vi "TestExec.Configure Local Station ID Read and Dialog.vi"(9 "Dialog":bool, 10 "Station":T1={"Name"="UNDEFINED", "PN"="UNDEFINED", "SN"="UNDEFINED", "Location"="UNDEFINED"}, 11 "Config File":path) -> (1 "Changed":bool, 3 "Station Out":T1)   [LabVIEW 2024]
uses:
  TestExec.Station ID.ctl
  <vilib>/Utility/config.llb/Read Key (String).vi
  <vilib>/Utility/config.llb/Write Key (String).vi
  <vilib>/Utility/config.llb/NI_LVConfig.lvlib
panel:
  out "Tab Control":enum32{"Inputs", "Data", "Outputs"}(tab)=enum."Data"
  in  "Default Sequence":u16(ring)
  in  "Additional Station  Config File":path
  in  "Changed":bool
  in  "Cancel":bool
  # "Local Station ID"
  # "(Optional)"
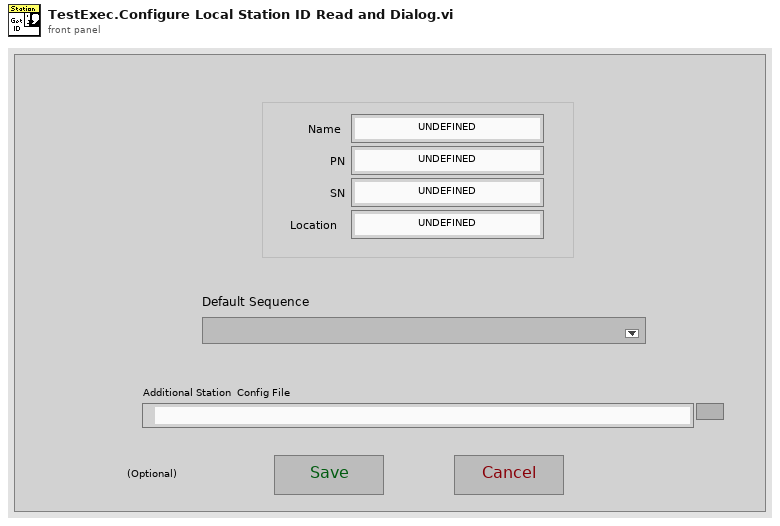
[diagram p1: front panel]
types:
  T1 = typedef "TestExec.Station ID.ctl" = cluster{"Name":string, "PN":string, "SN":string, "Location":string}
  T2 = enum32{"Invalid", "Standard", "Closed", "Hidden", "Minimized", "Maximized"}
  T3 = cluster{"Config File":path, "Changed":bool, "SeqDir":path}
  T4 = typedef "NI_LVConfig.lvlib/Config Data RefNum.ctl" = refnum<k1>
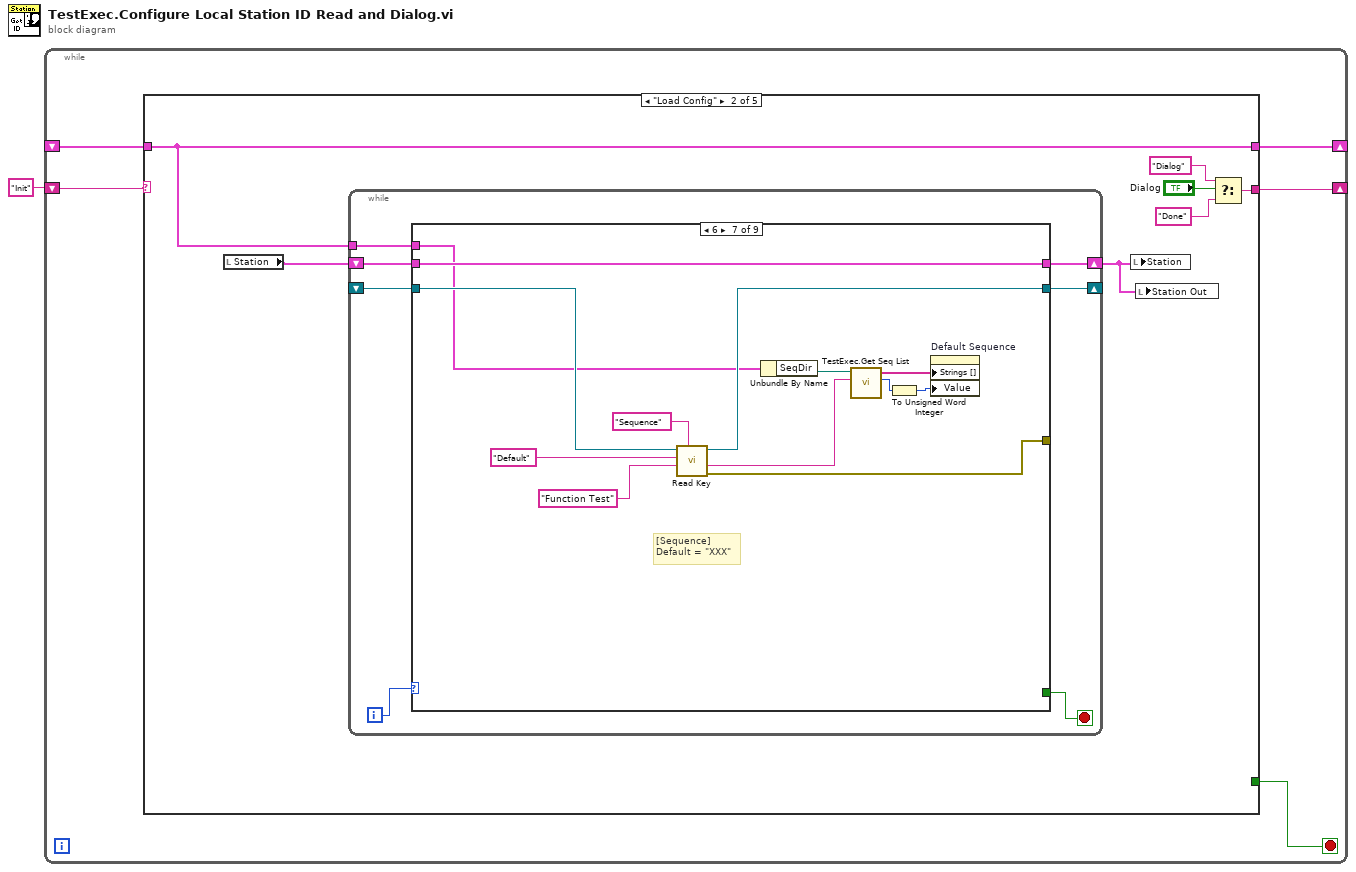
[diagram p0: block diagram]
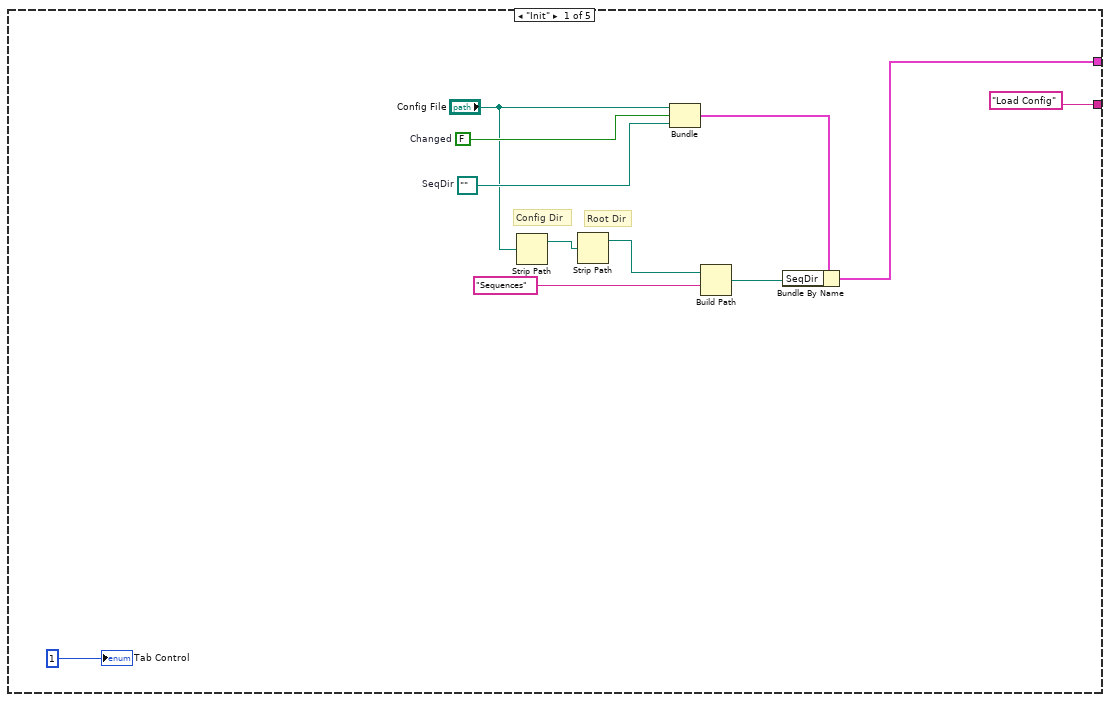
[diagram p2: hidden frame]
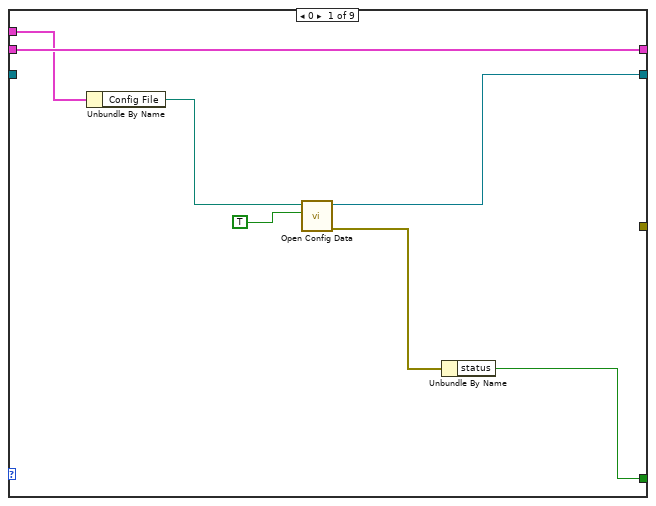
[diagram p3: hidden frame]
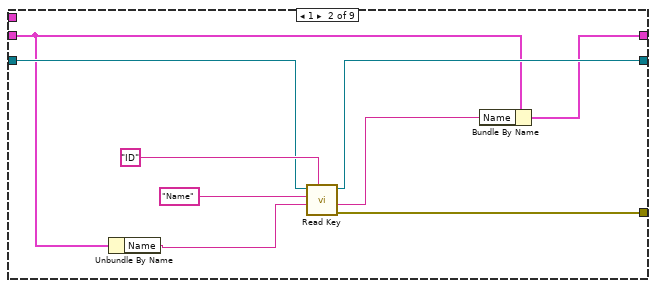
[diagram p4: hidden frame]
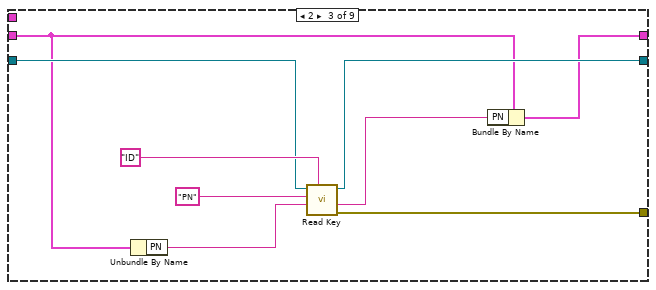
[diagram p5: hidden frame]
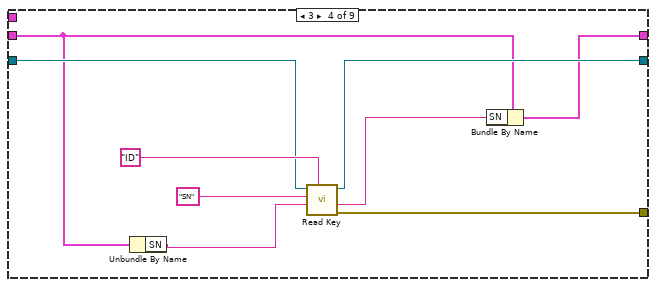
[diagram p6: hidden frame]
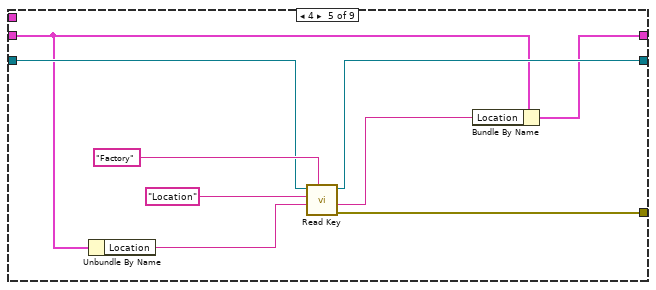
[diagram p7: hidden frame]
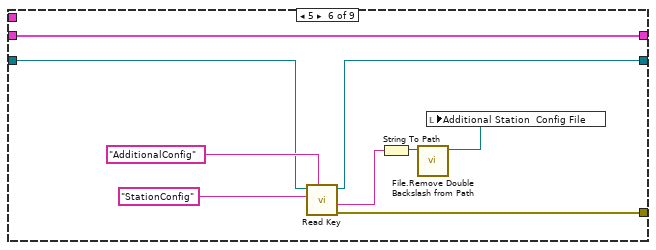
[diagram p8: hidden frame]
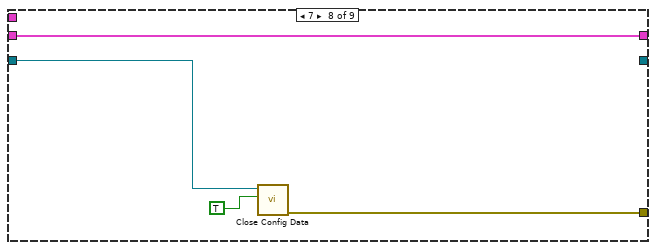
[diagram p9: hidden frame]
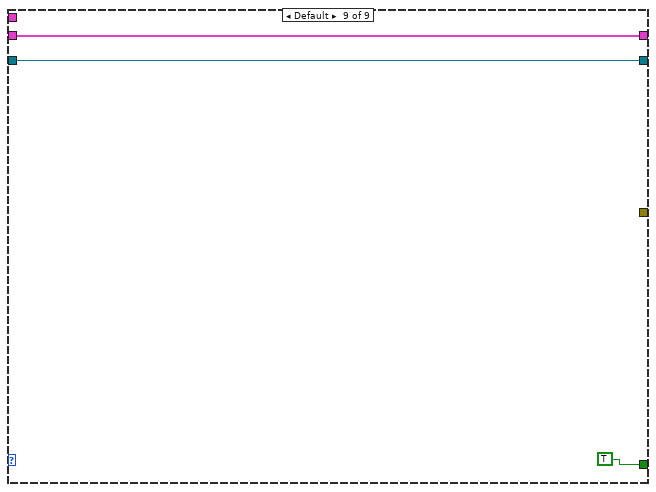
[diagram p10: hidden frame]
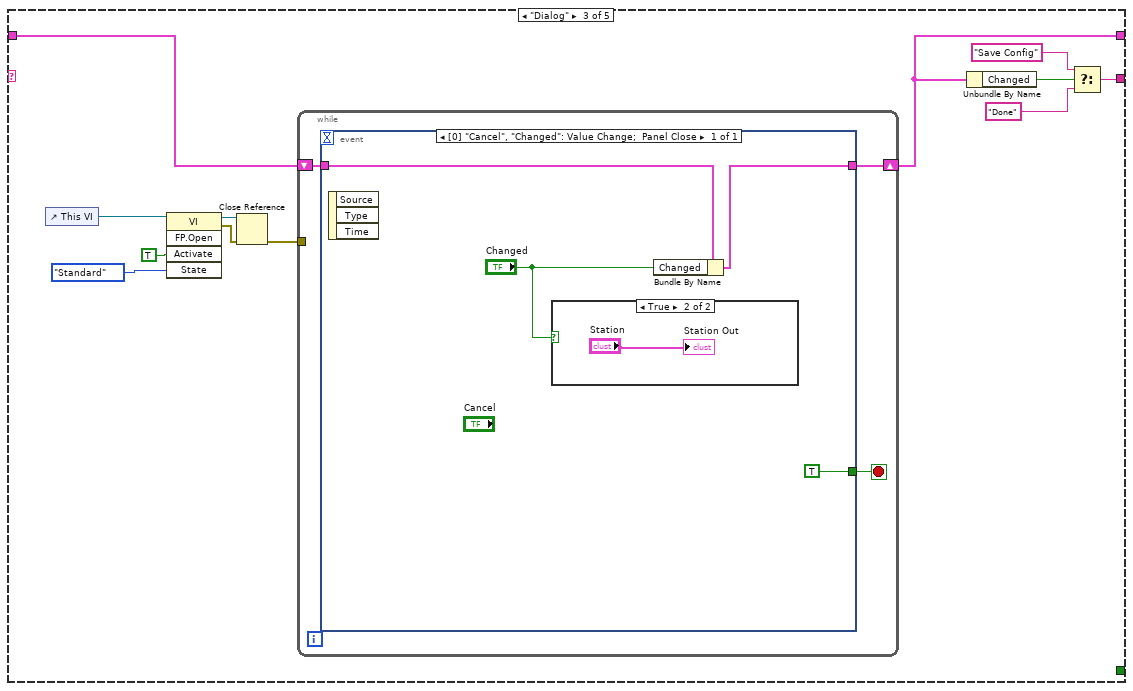
[diagram p11: hidden frame]
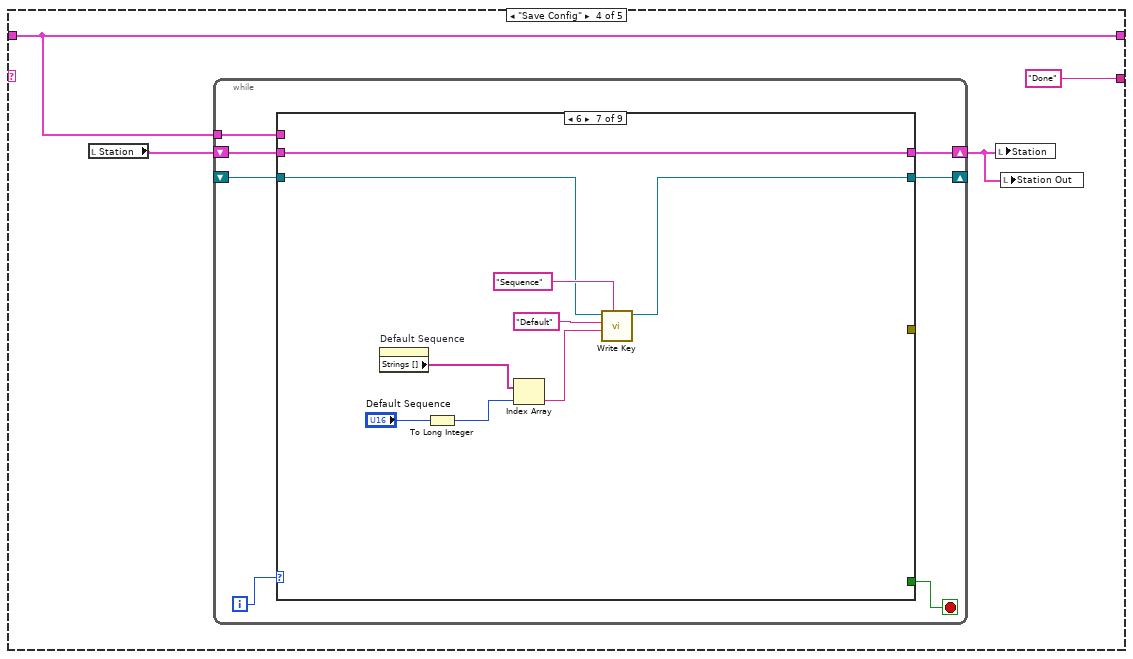
[diagram p13: hidden frame]
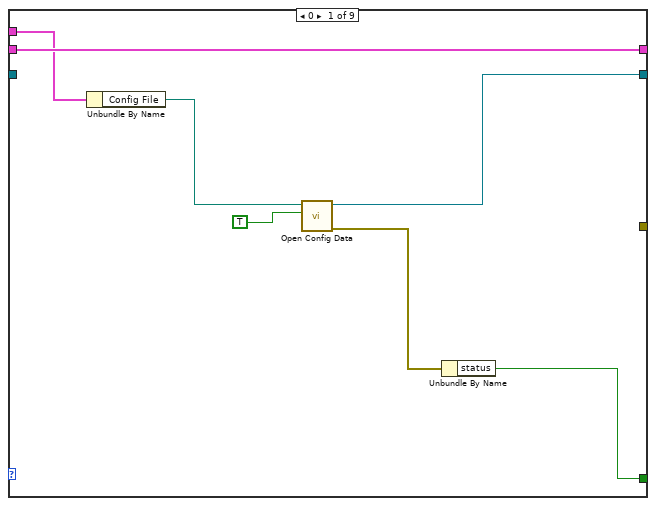
[diagram p14: hidden frame]
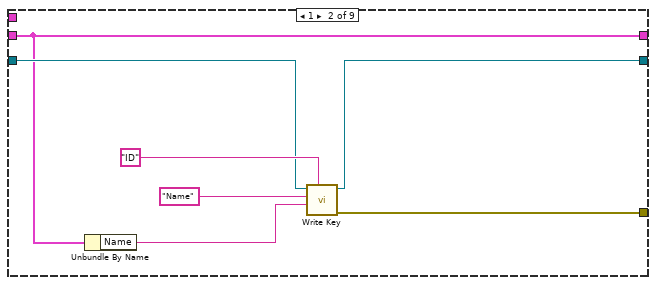
[diagram p15: hidden frame]
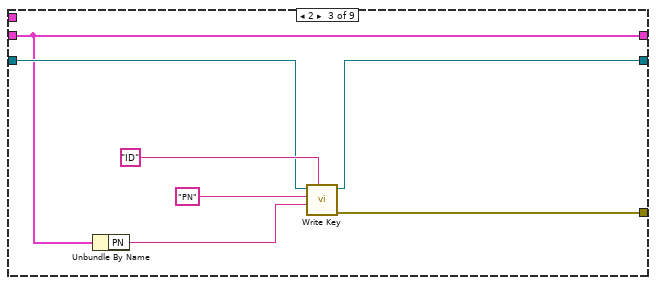
[diagram p16: hidden frame]
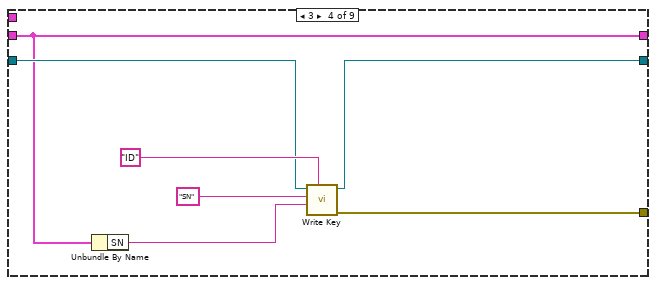
[diagram p17: hidden frame]
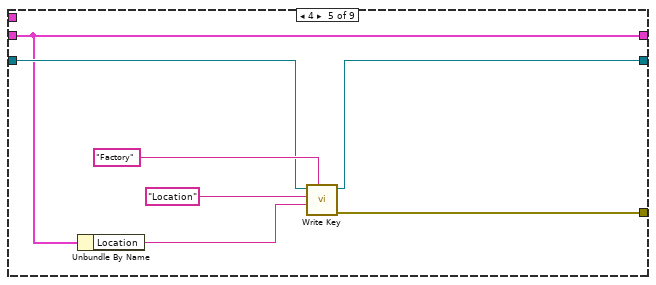
[diagram p18: hidden frame]
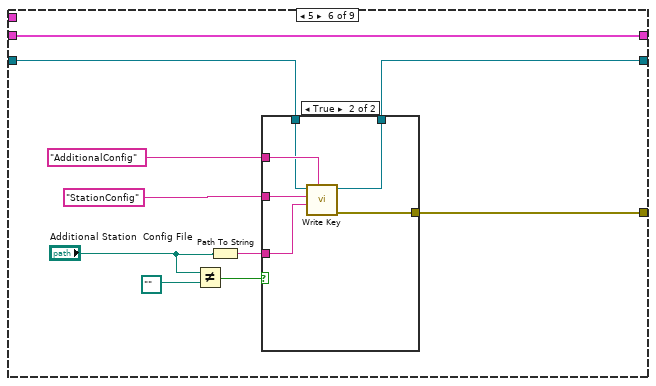
[diagram p19: hidden frame]
diagram:
  n1 = while {
    shift-right: [w4] -> _
    shift-left: _ -> [w6]
    shift-right: [w3] -> _
    shift-left: "Init" -> [w5]
    stop <- w2 stop-if-true
    n2 = case shown="\"Load Config\"" w5 {
      tunnel: w6 -> [_ w23 w109 w126 w207]
      tunnel: [w8 w23 w108 w126 w207] -> w4
      tunnel: ["Load Config" w21 w104 "Done" "Done"] -> w3
      tunnel: [_ _ _ _ TRUE] -> w2
      frame "Init" {
        w14 = path ""  # SeqDir
        w15 = FALSE  # Changed
        # "Root Dir"
        # "Config Dir"
        n3 = Strip Path(path="Config File") -> (stripped path=w11:path)  [unwired: 1 out]
        n4 = Strip Path(path=w11) -> (stripped path=w10:path)  [unwired: 1 out]
        n5 = Bundle("Config File"="Config File", "Changed"=w15, "SeqDir"=w14) -> (w9:T3)  [unwired: 1 in]
        n6 = Build Path(base path=w10, name or relative path="Sequences") -> (appended path=w7:path)
        n7 = Bundle By Name(cluster=w9, "SeqDir"=w7) -> (w8:T3)
        "Tab Control" <- 1
      }
      frame "Load Config" {
        n8 = local read "Station"() -> (w24:T1)
        n9 = while {
          shift-right: [w28] -> _
          shift-left: _ -> [w29]
          shift-right: [w27] -> w18
          shift-left: w24 -> [w26]
          tunnel: w23 -> [w25]
          i -> [w31]
          stop <- w30 stop-if-true
          n10 = case shown="6" w31 {
            tunnel: [w36 _ _ _ _ _ _ _ TRUE] -> w30
            tunnel: w29 -> [_ w44 w53 w62 w71 w80 w92 w100 w103]
            tunnel: [w38 w43 w52 w61 w70 w79 w93 _ w103] -> w28
            tunnel: [_ w47 w56 w65 w74 w83 w91 w99 _] -> _
            tunnel: [w34 w42 w51 w60 w69 w78 w96 w97 w102] -> w27
            tunnel: w26 -> [w34 w40 w49 w58 w67 w78 w96 w97 w102]
            tunnel: w25 -> [w33 _ _ _ _ _ w90 _ _]
            frame 0 {
              n11 = Unbundle By Name(w33) -> ("Config File"=w32:path)
              n12 = call <vilib>:"Open Config Data.vi"("create file if necessary (T)"=TRUE, "configuration file path"=w32) -> ("error out"=w37:errorcluster, "refnum"=w38:T4)  [unwired: 7 in, 1 out]
              n13 = Unbundle By Name(w37) -> ("status"=w36:bool)
            }
            frame 1 {
              n14 = Unbundle By Name(w40) -> ("Name"=w39:string)
              n15 = call-poly <vilib>:"Read Key.vi"("section"="ID", "default value"=w39, "key"="Name" ("section"), "refnum"=w44) -> ("error out"=w47:errorcluster, "value"=w41:string, "refnum out"=w43:T4)  [unwired: 4 in, 1 out]
              n16 = Bundle By Name(cluster=w40, "Name"=w41) -> (w42:T1)
            }
            frame 2 {
              n17 = Unbundle By Name(w49) -> ("PN"=w48:string)
              n18 = call-poly <vilib>:"Read Key.vi"("section"="ID", "default value"=w48, "key"="PN" ("section"), "refnum"=w53) -> ("error out"=w56:errorcluster, "value"=w50:string, "refnum out"=w52:T4)  [unwired: 4 in, 1 out]
              n19 = Bundle By Name(cluster=w49, "PN"=w50) -> (w51:T1)
            }
            frame 3 {
              n20 = Unbundle By Name(w58) -> ("SN"=w57:string)
              n21 = call-poly <vilib>:"Read Key.vi"("section"="ID", "default value"=w57, "key"="SN" ("section"), "refnum"=w62) -> ("error out"=w65:errorcluster, "value"=w59:string, "refnum out"=w61:T4)  [unwired: 4 in, 1 out]
              n22 = Bundle By Name(cluster=w58, "SN"=w59) -> (w60:T1)
            }
            frame 4 {
              n23 = Unbundle By Name(w67) -> ("Location"=w66:string)
              n24 = call-poly <vilib>:"Read Key.vi"("section"="Factory", "default value"=w66, "key"="Location" ("section"), "refnum"=w71) -> ("error out"=w74:errorcluster, "value"=w68:string, "refnum out"=w70:T4)  [unwired: 4 in, 1 out]
              n25 = Bundle By Name(cluster=w67, "Location"=w68) -> (w69:T1)
            }
            frame 5 {
              n26 = call-poly <vilib>:"Read Key.vi"("section"="AdditionalConfig", "key"="StationConfig" ("section"), "refnum"=w80) -> ("error out"=w83:errorcluster, "value"=w77:string, "refnum out"=w79:T4)  [unwired: 5 in, 1 out]
              n27 = String To Path(string=w77) -> (path=w76:path)
              n28 = call "File.Remove Double Backslash from Path.vi"("Path"=w76) -> ("Path Out"=w75:path)  [unwired: 10 in]
              n29 = local write "Additional Station  Config File"(w75) -> ()
            }
            frame 6 {
              # "[Sequence]\nDefault = \"XXX\""
              n30 = call-poly <vilib>:"Read Key.vi"("section"="Sequence", "default value"="Function Test", "key"="Default", "refnum"=w92) -> ("error out"=w91:errorcluster, "value"=w88:string, "refnum out"=w93:T4)  [unwired: 4 in, 1 out]
              n31 = Unbundle By Name(w90) -> ("SeqDir"=w89:path)
              n32 = call "TestExec.Get Seq List.vi"("DefaultSeq"=w88, "Seq Dir"=w89) -> ("Index"=w85:i32, "Seq List"=w87:string[])  [unwired: 8 in]
              n33 = To Unsigned Word Integer(number=w85) -> (unsigned 16bit integer=w86:u16)
              n34 = property on="Default Sequence" class="Ring (strict)"("Strings []"=w87, "Value"=w86) -> ()  [unwired: 2 in, 2 out]
            }
            frame 7 {
              n35 = call <vilib>:"Close Config Data.vi"("write file if changed (T)"=TRUE, "refnum"=w100) -> ("error out"=w99:errorcluster)  [unwired: 8 in, 1 out]
            }
            frame Default {
            }
          }
        }
        n36 = local write "Station"(w18) -> ()
        n37 = local write "Station Out"(w18) -> ()
        n38 = Select(t="Dialog", s="Dialog", f="Done") -> (s? t:f=w21:string)
      }
      frame "Dialog" {
        n39 = control-ref of="This VI"() -> (w115:refnum<vi>)
        n40 = invoke class="VI" method="FP.Open"(reference=w115, "Activate"=TRUE ("Activate?"), "State"=T2."Standard") -> (reference out=w112:refnum<vi>, error out=w111:errorcluster)  [unwired: 2 in, 3 out]
        n41 = Close Reference(reference=w112, error in (no error)=w111) -> (error out=w110:errorcluster)
        n42 = while {
          tunnel: w110 -> [_]
          shift-right: [w116] -> w108
          shift-left: w109 -> [w117]
          stop <- w118 stop-if-true
          n43 = event shown="[0] \"Cancel\", \"Changed\": Value Change;  Panel Close" {
            selector: _ -> [_]
            dyn-events: _ -> [_]
            timeout: _ -> [_]
            tunnel: [TRUE] -> w118
            tunnel: w117 -> [w121]
            tunnel: [w120] -> w116
            event "Cancel", "Changed": Value Change; Panel Close {
              n44 = event-data() -> ()  [unwired: 1 in, 3 out]
              n45 = case shown="True" "Changed" {
                frame False {
                }
                frame True {
                  "Station Out" <- "Station"
                }
              }
              n46 = Bundle By Name(cluster=w121, "Changed"="Changed") -> (w120:T3)
            }
          }
        }
        n47 = Unbundle By Name(w108) -> ("Changed"=w107:bool)
        n48 = Select(t="Save Config", s=w107, f="Done") -> (s? t:f=w104:string)
      }
      frame "Save Config" {
        n49 = local read "Station"() -> (w127:T1)
        n50 = while {
          shift-right: [w131] -> _
          shift-left: _ -> [w132]
          shift-right: [w130] -> w125
          shift-left: w127 -> [w129]
          tunnel: w126 -> [w128]
          i -> [w134]
          stop <- w133 stop-if-true
          n51 = case shown="6" w134 {
            tunnel: [w139 _ _ _ _ _ _ _ TRUE] -> w133
            tunnel: w132 -> [_ w145 w152 w159 w166 w176 w191 w199 w202]
            tunnel: [w141 w144 w151 w158 w165 w175 w192 _ w202] -> w131
            tunnel: [_ w148 w155 w162 w169 w179 _ w198 _] -> _
            tunnel: [w137 w142 w149 w156 w163 w174 w195 w196 w201] -> w130
            tunnel: w129 -> [w137 w142 w149 w156 w163 w174 w195 w196 w201]
            tunnel: w128 -> [w136 _ _ _ _ _ _ _ _]
            frame 0 {
              n52 = Unbundle By Name(w136) -> ("Config File"=w135:path)
              n53 = call <vilib>:"Open Config Data.vi"("create file if necessary (T)"=TRUE, "configuration file path"=w135) -> ("error out"=w140:errorcluster, "refnum"=w141:T4)  [unwired: 7 in, 1 out]
              n54 = Unbundle By Name(w140) -> ("status"=w139:bool)
            }
            frame 1 {
              n55 = Unbundle By Name(w142) -> ("Name"=w143:string)
              n56 = call-poly <vilib>:"Write Key.vi"("section"="ID", "value"=w143, "key"="Name" ("section"), "refnum"=w145) -> ("error out"=w148:errorcluster, "refnum out"=w144:T4)  [unwired: 5 in, 1 out]
            }
            frame 2 {
              n57 = Unbundle By Name(w149) -> ("PN"=w150:string)
              n58 = call-poly <vilib>:"Write Key.vi"("section"="ID", "value"=w150, "key"="PN" ("section"), "refnum"=w152) -> ("error out"=w155:errorcluster, "refnum out"=w151:T4)  [unwired: 5 in, 1 out]
            }
            frame 3 {
              n59 = Unbundle By Name(w156) -> ("SN"=w157:string)
              n60 = call-poly <vilib>:"Write Key.vi"("section"="ID", "value"=w157, "key"="SN" ("section"), "refnum"=w159) -> ("error out"=w162:errorcluster, "refnum out"=w158:T4)  [unwired: 5 in, 1 out]
            }
            frame 4 {
              n61 = Unbundle By Name(w163) -> ("Location"=w164:string)
              n62 = call-poly <vilib>:"Write Key.vi"("section"="Factory", "value"=w164, "key"="Location" ("section"), "refnum"=w166) -> ("error out"=w169:errorcluster, "refnum out"=w165:T4)  [unwired: 5 in, 1 out]
            }
            frame 5 {
              n63 = Not Equal?(x="Additional Station  Config File", y=path "") -> (x != y?=w172:bool)
              n64 = Path To String(path="Additional Station  Config File") -> (string=w170:string)
              n65 = case shown="True" w172 {
                tunnel: [_ w186] -> w179
                tunnel: "AdditionalConfig" ("section") -> [_ w185]
                tunnel: "StationConfig" ("section") -> [_ w184]
                tunnel: w176 -> [w180 w183]
                tunnel: [w180 w182] -> w175
                tunnel: w170 -> [_ w181]
                frame False {
                }
                frame True {
                  n66 = call-poly <vilib>:"Write Key.vi"("section"=w185, "value"=w181, "key"=w184, "refnum"=w183) -> ("error out"=w186:errorcluster, "refnum out"=w182:T4)  [unwired: 5 in, 1 out]
                }
              }
            }
            frame 6 {
              n67 = property on="Default Sequence" class="Ring (strict)"() -> ("Strings []"=w190:string[])  [unwired: 2 in, 2 out]
              n68 = To Long Integer(number="Default Sequence") -> (32bit integer=w187:i32)
              n69 = Index Array(array=w190, index=w187) -> (element=w189:string)
              n70 = call-poly <vilib>:"Write Key.vi"("section"="Sequence", "value"=w189, "key"="Default" ("section"), "refnum"=w191) -> ("refnum out"=w192:T4)  [unwired: 5 in, 2 out]
            }
            frame 7 {
              n71 = call <vilib>:"Close Config Data.vi"("write file if changed (T)"=TRUE, "refnum"=w199) -> ("error out"=w198:errorcluster)  [unwired: 8 in, 1 out]
            }
            frame Default {
            }
          }
        }
        n72 = local write "Station"(w125) -> ()
        n73 = local write "Station Out"(w125) -> ()
      }
      frame "Done", Default {
        w204 = TRUE  # Normal(T)/Debug(F)
        n74 = Unbundle By Name(w207) -> ("Changed"=→"Changed":bool)
        n75 = local read "Dialog"() -> (w205:bool)
        n76 = And(x=w205, y=w204) -> (x .and. y?=w203:bool)
        n77 = case shown="True" w203 {
          tunnel: [_ w210] -> _
          frame False {
          }
          frame True {
            n78 = control-ref of="This VI"() -> (w213:refnum<vi>)
            n79 = invoke class="VI" method="FP.Close"(reference=w213) -> (reference out=w212:refnum<vi>, error out=w211:errorcluster)  [unwired: 2 in, 1 out]
            n80 = Close Reference(reference=w212, error in (no error)=w211) -> (error out=w210:errorcluster)
          }
        }
      }
    }
  }
